vi "uncertainty_datasets.vi"(4 "Discesa":dbl[][](array[numeric]), 7 "Salita":dbl[][](array[numeric])) -> (0 "uncertainty ascending phase (point-by-point)":dbl[](array[numeric]), 1 "uncertainty descending phase (point-by-point)":dbl[](array[numeric]), 2 "Maximum uncertainty Descending Phase":dbl, 3 "Maximum uncertainty Ascending Phase":dbl)   [LabVIEW 2021, in "CALIBRATION.lvlib"]
uses:
  CALIBRATION.lvlib
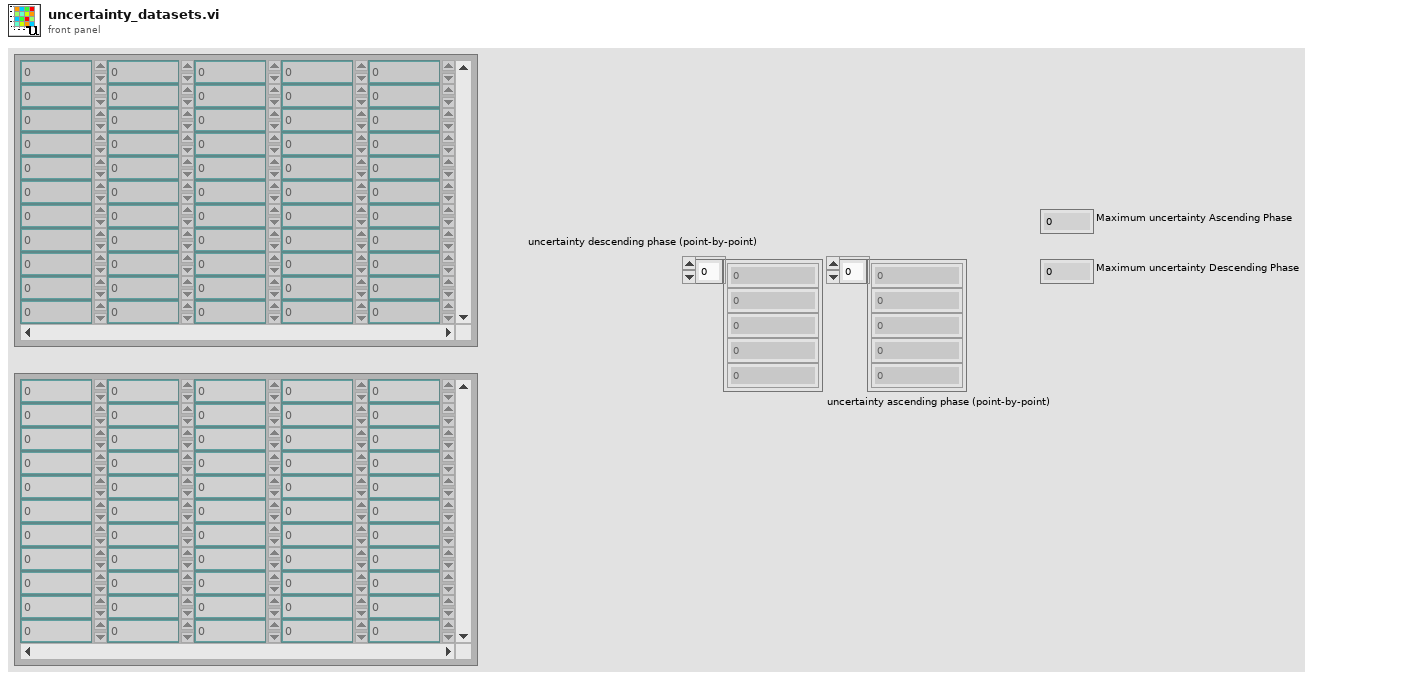
[diagram p1: front panel]
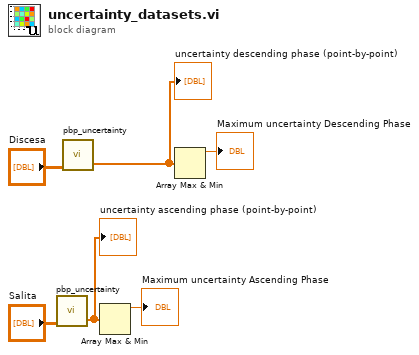
[diagram p0: block diagram]
diagram:
  n1 = call "pbp_uncertainty.vi"("insieme"="Salita") -> ("Incertezza"=w2:dbl[])  [unwired: 4 in]
  "uncertainty ascending phase (point-by-point)" <- w2
  n2 = call "pbp_uncertainty.vi"("insieme"="Discesa") -> ("Incertezza"=w1:dbl[])  [unwired: 4 in]
  "uncertainty descending phase (point-by-point)" <- w1
  n3 = Array Max & Min(array=w2) -> (max value=→"Maximum uncertainty Ascending Phase":dbl)  [unwired: 3 out]
  n4 = Array Max & Min(array=w1) -> (max value=→"Maximum uncertainty Descending Phase":dbl)  [unwired: 3 out]
